vi "Post-Project-Copying Process - Error Handling.vi"(8 "error in":errorcluster) -> (0 "error out":errorcluster)   [LabVIEW 2021, in "LV Scripting Utilities.lvlib"]
uses:
  LV Scripting Utilities.lvlib
  <vilib>/Utility/error.llb/DialogType.ctl
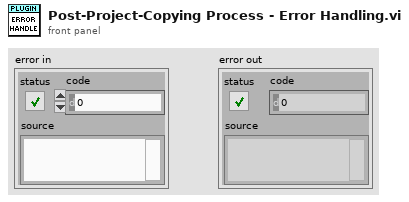
[diagram p1: front panel]
types:
  T1 = typedef "DialogType.ctl" = u16
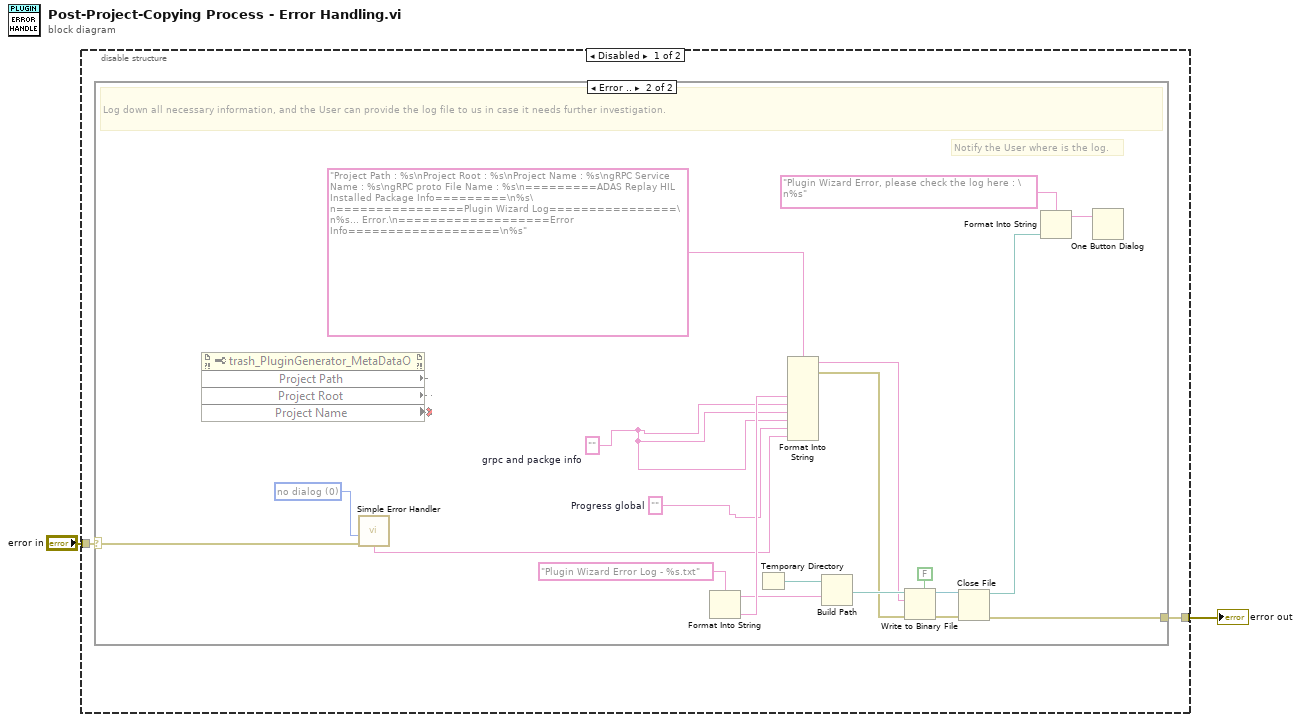
[diagram p0: block diagram]
diagram:
  n1 = disable-structure shown="Disabled" {
    disable-tunnel: [w4 _] -> w2
    disable-tunnel: "error in" -> [w3 _]
    frame Disabled {
      n2 = case shown="Error .." w3 {
        selector: w3 -> [w5 w27]
        tunnel: [w5 w10] -> w4
        frame No Error {
        }
        frame Error {
          w6 = ""  # Progress global
          w7 = ""  # grpc and packge info
          w26 = T1 0 items=["no dialog", "OK message", "continue or stop message", "OK message + warnings", "continue/stop + warnings"] ("type of dialog (OK msg:1)")
          # "Notify the User where is the log."
          # "Log down all necessary information, and the User can provide the log file to us in case it needs further investigation."
          n3 = call <vilib>:"Simple Error Handler.vi"("type of dialog (OK msg:1)"=w26, "error in (no error)"=w27) -> ("message"=w8:string)  [unwired: 3 in, 4 out]
          n4 = Temporary Directory() -> (w22:path)
          n5 = Format Into String(format string="Project Path : %s\nProject Root : %s\nProject Name : %s\ngRPC Service Name : %s\ngRPC proto File Name : %s\n=========ADAS Replay HIL Installed Package Info=========\n%s\n================Plugin Wizard Log================\n%s... Error.\n===================Error Info===================\n%s", w7, w7, w7, w6, w8) -> (resulting string=w17:string, error out=w16:errorcluster, w25:path, w24:path, w21:string)  [unwired: 2 in]
          n6 = Format Into String(format string="Plugin Wizard Error Log - %s.txt", w21) -> (resulting string=w19:string)  [unwired: 2 in, 1 out]
          n7 = Build Path(base path=w22, name or relative path=w19) -> (appended path=w18:path)
          n8 = Write to Binary File(file (use dialog)=w18, data=w17, error in=w16, 5:FALSE ("prepend array or string size? (T)")) -> (refnum out=w14:refnum<file>, error out=w15:errorcluster)  [unwired: 2 in, 1 out]
          n9 = Close File(refnum=w14, error in=w15) -> (path=w13:path, error out=w10:errorcluster)
          n10 = Format Into String(format string="Plugin Wizard Error, please check the log here : \n%s", w13) -> (resulting string=w11:string)  [unwired: 2 in, 1 out]
          n11 = One Button Dialog(message=w11) -> ()  [unwired: 1 in, 1 out]
        }
      }
    }
    frame Enabled {
    }
  }
  "error out" <- w2
